vi "rack_info.vi"() -> ()   [LabVIEW 2014]
uses:
  <vilib>/Easy HTTP Client/Easy HTTP.lvlib
panel:
  out "Response":string
  in  "Host":string
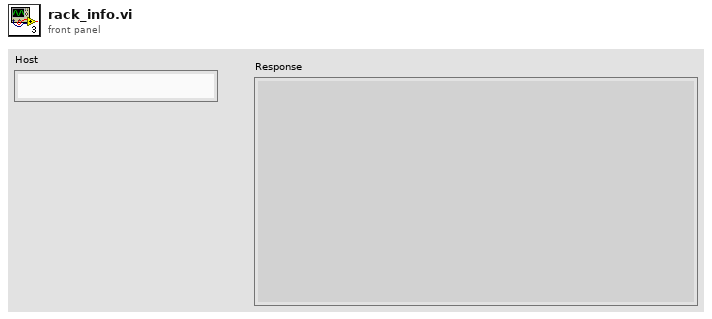
[diagram p1: front panel]
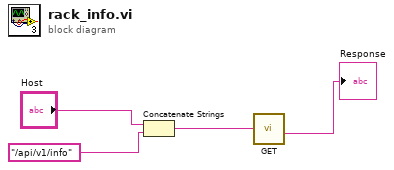
[diagram p0: block diagram]
diagram:
  n1 = Concatenate Strings("Host", "/api/v1/info") -> (w1:string)
  n2 = call <vilib>:"GET.vi"("url"=w1) -> ("body"=→"Response":string)  [unwired: 6 in, 4 out]
